vi "StructureToJson.vi"(6 "Component Idx":i32, 7 "Relative Bounds":cluster{"x":i32, "y":i32, "w":i32, "h":i32}, 8 "error in (no error)":errorcluster, 9 "Origin Path":path, 10 "Current Path":path, 11 "GObj (in)":refnum<vi>) -> (0 "error out":errorcluster, 3 "JSON":string)   [LabVIEW 2017]
doc: "Creates a JSON for a structure"
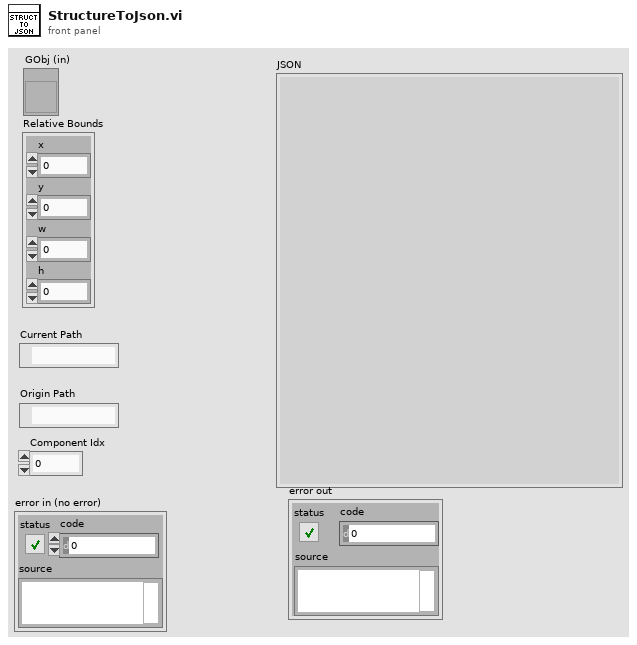
[diagram p1: front panel]
types:
  T1 = typedef "LVRectTypeDef.ctl" = cluster{"Left":i16, "Top":i16, "Right":i16, "Bottom":i16}
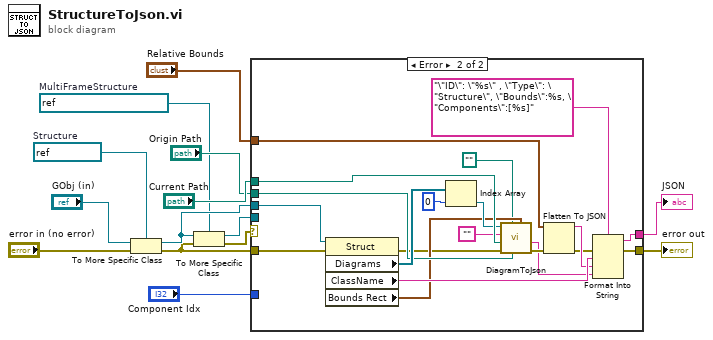
[diagram p0: block diagram]
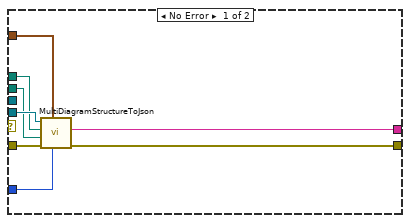
[diagram p2: hidden frame]
diagram:
  w4 = refnum<vi> refnum  # MultiFrameStructure
  w14 = refnum<vi> refnum  # Structure
  n1 = To More Specific Class(target class=w14, reference="GObj (in)", error in="error in (no error)") -> (specific class reference=w5:refnum<vi>, error out=w1:errorcluster)
  n2 = To More Specific Class(target class=w4, reference=w5, error in=w1) -> (specific class reference=w3:refnum<vi>, error out=w2:errorcluster)
  n3 = case shown="Error" w2 {
    tunnel: "Current Path" -> [w21 w42]
    tunnel: "Component Idx" -> [w19 _]
    tunnel: w5 -> [_ w41]
    tunnel: [w16 w35] -> w9
    tunnel: "Origin Path" -> [w20 w34]
    tunnel: [w17 w30] -> w8
    tunnel: "Relative Bounds" -> [w15 w33]
    tunnel: w1 -> [w18 w23]
    tunnel: w3 -> [w22 _]
    frame No Error {
      n4 = call "MultiDiagramStructureToJson.vi"("Component Idx"=w19, "Relative Bounds"=w15, "error in (no error)"=w18, "Origin Path"=w20, "Current Path"=w21, "MultiDiagramStructure in"=w22) -> ("error out"=w17:errorcluster, "JSON"=w16:string)  [unwired: 4 in]
    }
    frame Error {
      n5 = property class="Struct"(reference=w41, error in=w23) -> (error out=w25:errorcluster, "Diagrams"=w40:refnum<vi>[], "ClassName"=w36:string, "Bounds Rect"=w31:T1)  [unwired: 1 out]
      n6 = Index Array(array=w40, index=0) -> (element=w38:refnum<vi>)
      n7 = call "DiagramToJson.vi"("Owner Bounds"=w31, "Origin Path"=w34, "Image Path"=path "", "error in (no error)"=w25, "Current Path"=w42, "ID"="", "GObj in"=w38) -> ("error out"=w28:errorcluster, "JSON (out)"=w26:string)  [unwired: 2 in, 1 out]
      n8 = Flatten To JSON(anything=w33, error in (no error)=w28) -> (JSON string=w32:string, 11:w27:errorcluster)  [unwired: 1 in]
      n9 = Format Into String(format string="\"ID\": \"%s\" , \"Type\": \"Structure\", \"Bounds\":%s, \"Components\":[%s]", error in=w27, w36, w32, w26) -> (resulting string=w35:string, error out=w30:errorcluster)  [unwired: 1 in]
    }
  }
  "JSON" <- w9
  "error out" <- w8
